vi "AI@Export2COCO__Parameter.vi"(1 "ParamterIn":string) -> (0 "ParamterOut":string)   [LabVIEW 2020]
uses:
  MainFrame/Global.vi
  <vilib>/vision/NI_Vision_Development_Module.lvlib
panel:
  out "start":i32
  out "f":i32
  in  "CoCoFile":string(combo)
  out "Image":T1(plugin-control)
  in  "Preview":bool
  in  "SubDir":string(combo)
  in  "Capture":string(combo)
  in  "Confirm":bool
  # "AI@Export2COCO $Capture(\\$Directory),$CoCo.json"
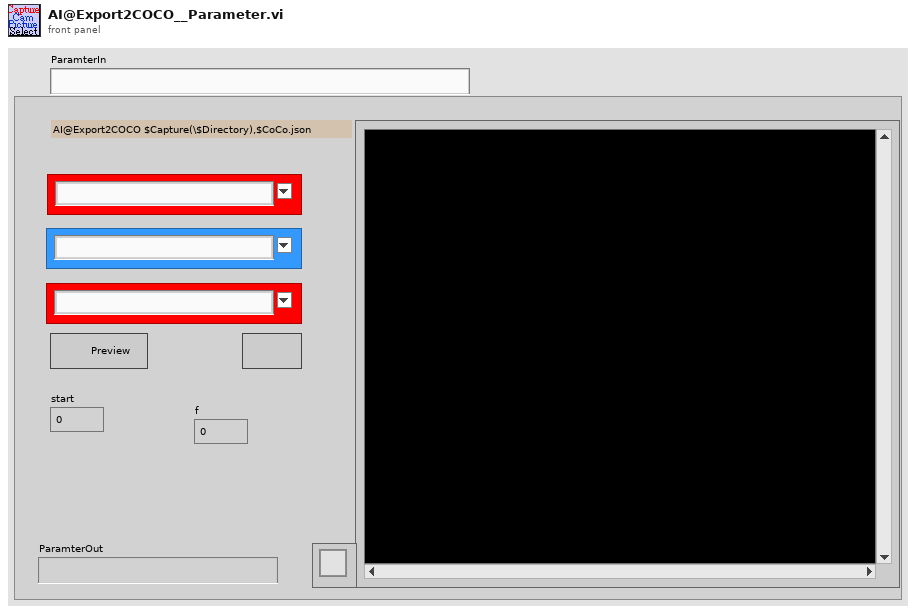
[diagram p1: front panel]
types:
  T1 = typedef "IMAQ Image.ctl" = refnum<image>
  T2 = cluster{"Browser Size":cluster{"X":i32, "Y":i32}, "Images per Line":i32, "Background Color":u32, "Frame Size":i32, "Frame Style":u16}
  T3 = typedef "Image Type" = u32
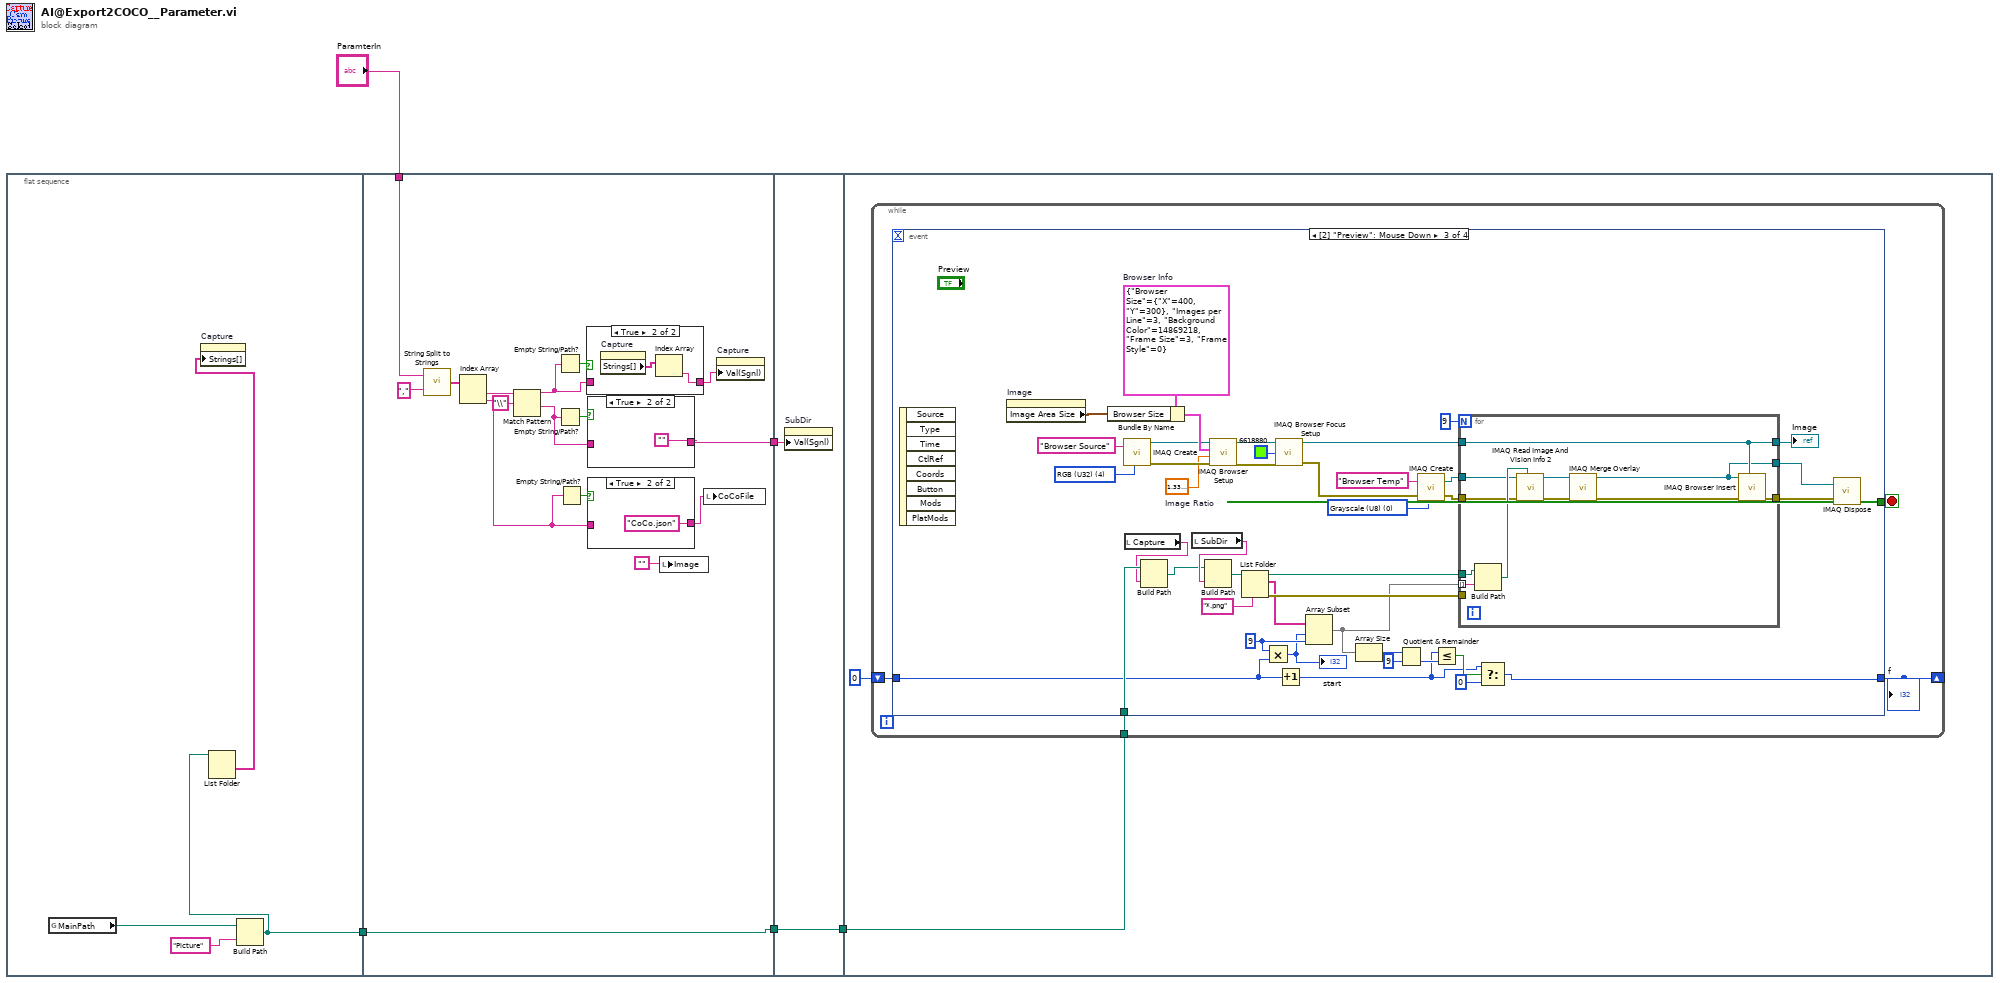
[diagram p0: block diagram]
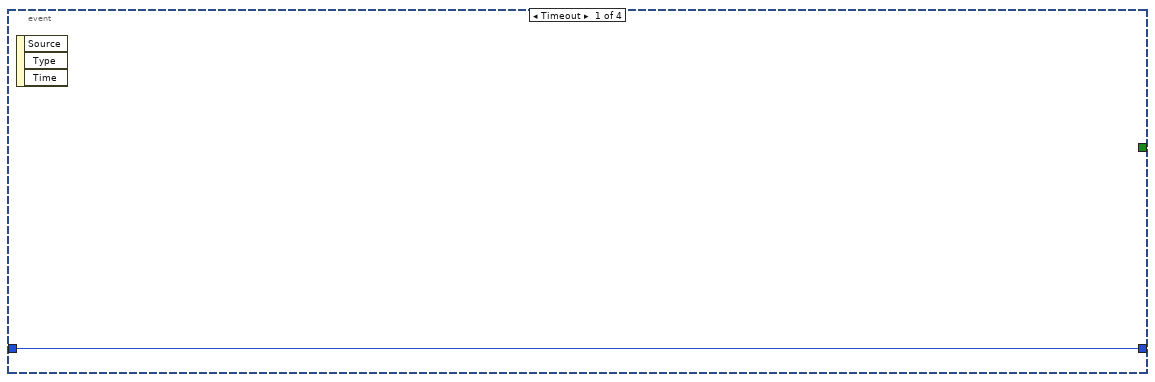
[diagram p5: hidden frame]
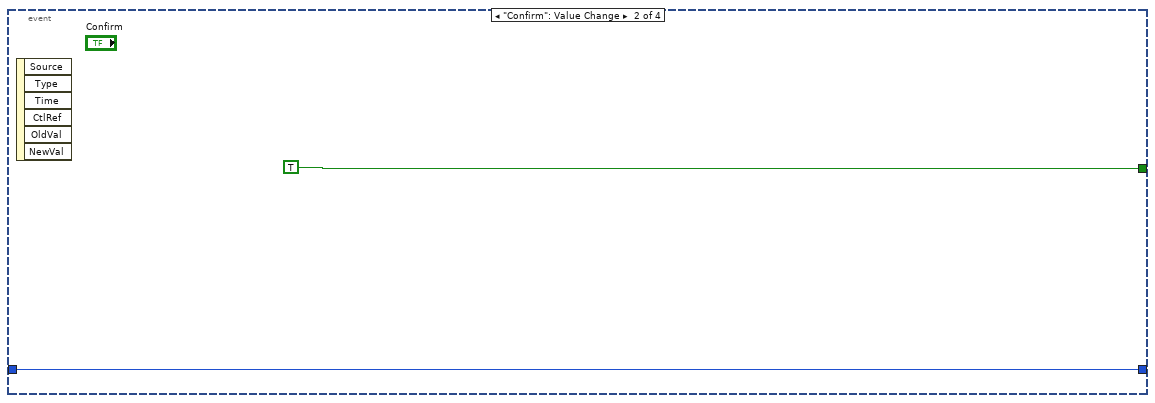
[diagram p6: hidden frame]
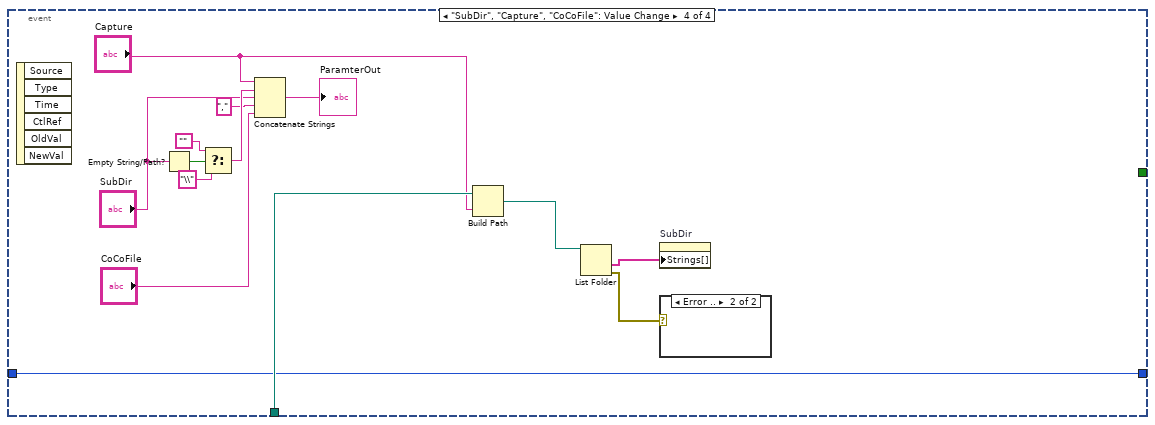
[diagram p7: hidden frame]
diagram:
  n1 = flat-sequence {
    tunnel: [w7] -> w2
    tunnel: "ParamterIn" -> [w23]
    tunnel: [w21] -> w3
    tunnel: w2 -> [w21]
    tunnel: [w20] -> w1
    tunnel: [w34] -> w4
    tunnel: w3 -> [w34]
    tunnel: w1 -> [w33]
    tunnel: w4 -> [w36]
    frame #0 {
      n2 = global read "Global.vi" "MainPath"() -> (w8:path)
      n3 = Build Path(base path=w8, name or relative path="Picture") -> (appended path=w7:path)
      n4 = List Folder(path=w7) -> (folder names=w6:string[])  [unwired: 3 in, 3 out]
      n5 = property on="Capture" class="CmbBox"("Strings[]"=w6) -> ()  [unwired: 2 in, 2 out]
    }
    frame #1 {
      n6 = call "String Split to Strings.vi"("search string/char (-)"=",", "String"=w23) -> ("Array"=w25:string[])
      n7 = Index Array(array=w25) -> (element #1=w17:string, element #2=w10:string)  [unwired: 2 in]
      n8 = Match Pattern(string=w17, regular expression="\\") -> (before substring=w15:string, after substring=w14:string)  [unwired: 1 in, 2 out]
      n9 = Empty String/Path?(string/path=w15) -> (empty?=w22:bool)
      n10 = Empty String/Path?(string/path=w14) -> (empty?=w18:bool)
      n11 = Empty String/Path?(string/path=w10) -> (empty?=w11:bool)
      n12 = case shown="True" w22 {
        tunnel: w15 -> [w30 _]
        tunnel: [w30 w31] -> w19
        frame False {
        }
        frame True {
          n13 = property on="Capture" class="CmbBox"() -> ("Strings[]"=w32:string[])  [unwired: 2 in, 2 out]
          n14 = Index Array(array=w32) -> (element=w31:string)  [unwired: 1 in]
        }
      }
      n15 = case shown="True" w18 {
        tunnel: [w28 ""] -> w20
        tunnel: w14 -> [w28 _]
        frame False {
        }
        frame True {
        }
      }
      n16 = case shown="True" w11 {
        tunnel: [w26 "CoCo.json"] -> w12
        tunnel: w10 -> [w26 _]
        frame False {
        }
        frame True {
        }
      }
      n17 = local write "Image"("") -> ()
      n18 = local write "CoCoFile"(w12) -> ()
      n19 = property on="Capture" class="CmbBox"("Val(Sgnl)"=w19) -> ()  [unwired: 2 in, 2 out]
    }
    frame #2 {
      n20 = property on="SubDir" class="CmbBox"("Val(Sgnl)"=w33) -> ()  [unwired: 2 in, 2 out]
    }
    frame #3 {
      n21 = while {
        tunnel: w36 -> [w39]
        shift-right: [w37] -> _
        shift-left: 0 -> [w38]
        stop <- w40 stop-if-true
        n22 = event shown="[2] \"Preview\": Mouse Down" {
          selector: _ -> [_ _ _ _]
          dyn-events: _ -> [_ _ _ _]
          timeout: _ -> [_ _ _ _]
          tunnel: [_ TRUE _ _] -> w40
          tunnel: w39 -> [_ _ w59 w107]
          tunnel: w38 -> [w41 w42 w53 w96]
          tunnel: [w41 w42 w45 w96] -> w37
          event Timeout {
            n23 = event-data() -> ()  [unwired: 1 in, 3 out]
          }
          event "Confirm": Value Change {
            n24 = event-data() -> ()  [unwired: 1 in, 6 out]
          }
          event "Preview": Mouse Down {
            w55 = 9 ("length")
            w63 = sgl 1.33  # Image Ratio
            w80 = T2 {"Browser Size"={"X"=400, "Y"=300}, "Images per Line"=3, "Background Color"=14869218, "Frame Size"=3, "Frame Style"=0}  # Browser Info
            w71 = T3 0 items=["Grayscale (U8)", "Grayscale (I16)", "Grayscale (SGL)", "Complex (CSG)", "RGB (U32)", "HSL (U32)", "RGB (U64)", "Grayscale (U16)"] ("Image Type")
            w69 = T3 4 items=["Grayscale (U8)", "Grayscale (I16)", "Grayscale (SGL)", "Complex (CSG)", "RGB (U32)", "HSL (U32)", "RGB (U64)", "Grayscale (U16)"] ("Image Type")
            n25 = event-data() -> ()  [unwired: 1 in, 8 out]
            n26 = property on="Image" class="ImageControl"() -> ("Image Area Size"=w81:cluster{"Width":u32, "Height":u32})  [unwired: 2 in, 2 out]
            n27 = Bundle By Name(cluster=w80, "Browser Size"=w81) -> (w82:T2)
            n28 = call "IMAQ Create"("Image Name"="Browser Source", "Image Type"=w69) -> ("New Image"=w67:T1, "error out"=w68:errorcluster)  [unwired: 3 in]
            n29 = local read "Capture"() -> (w58:string)
            n30 = Build Path(base path=w59, name or relative path=w58) -> (appended path=w57:path)
            n31 = local read "SubDir"() -> (w62:string)
            n32 = Build Path(base path=w57, name or relative path=w62) -> (appended path=w61:path)
            n33 = call "IMAQ Browser Setup"("error in (no error)"=w68, "Image Ratio"=w63, "Browser Info"=w82, "Image In"=w67) -> ("error out"=w76:errorcluster, "Image Browser Out"=w75:T1)  [unwired: 2 out]
            n34 = List Folder(path=w61, pattern="*.png") -> (path out=w66:path, filenames=w44:string[], error out=w83:errorcluster)  [unwired: 2 in, 1 out]
            n35 = Multiply(x=w55, y=w53) -> (x*y=w54:i32)
            "start" <- w54
            n36 = call "IMAQ Browser Focus Setup"("error in (no error)"=w76, "Focus Color"=u32 6618880, "Image Browser In"=w75) -> ("error out"=w78:errorcluster, "Image Browser Out"=w77:T1)  [unwired: 1 in]
            n37 = Increment(x=w53) -> (x+1=w47:i32)
            n38 = Array Subset(array=w44, index=w54, length=w55) -> (w52:string[])
            n39 = Array Size(array=w52) -> (size(s)=w51:i32)
            n40 = Quotient & Remainder(x=w51, y=9) -> (floor(x/y)=w49:i32)  [unwired: 1 out]
            n41 = call "IMAQ Create"("Image Name"="Browser Temp", "Image Type"=w71, "error in (no error)"=w78) -> ("New Image"=w73:T1, "error out"=w64:errorcluster)  [unwired: 2 in]
            n42 = Less Or Equal?(x=w47, y=w49) -> (x <= y?=w48:bool)
            n43 = for {
              N: 9 -> [_]
              tunnel: w77 -> [w90]
              tunnel: w66 -> [w95]
              tunnel: w64 -> [w93]
              tunnel: [w92] -> w65
              tunnel: [w90] -> w84
              tunnel: w73 -> [w91]
              tunnel: [w87] -> w74
              tunnel: w83 -> [_]
              tunnel: w52 -> [w85] mode=indexing
              n44 = Build Path(base path=w95, name or relative path=w85) -> (appended path=w94:path)
              n45 = call "IMAQ Read Image And Vision Info 2"("File Path"=w94, "error in (no error)"=w93, "Image"=w91) -> ("error out"=w89:errorcluster, "Image Out"=w88:T1)  [unwired: 6 in, 1 out]
              n46 = call "IMAQ Merge Overlay"("error in (no error)"=w89, "Image Src"=w88) -> ("error out"=w86:errorcluster, "Image Dst Out"=w87:T1)  [unwired: 8 in]
              n47 = call "IMAQ Browser Insert"("Image Browser In"=w90, "error in (no error)"=w86, "Image to Add"=w87) -> ("error out"=w92:errorcluster)  [unwired: 4 in, 4 out]
            }
            "Image" <- w84
            n48 = Select(t=w47, s=w48, f=0) -> (s? t:f=w45:i32)
            n49 = call "IMAQ Dispose"("Image"=w74, "error in (no error)"=w65) -> ()  [unwired: 4 in, 1 out]
          }
          event "SubDir", "Capture", "CoCoFile": Value Change {
            n50 = event-data() -> ()  [unwired: 1 in, 6 out]
            n51 = Empty String/Path?(string/path="SubDir") -> (empty?=w103:bool)
            n52 = Select(t="", s=w103, f="\\" ("string")) -> (s? t:f=w100:string)
            n53 = Concatenate Strings("Capture", w100, "SubDir", "," ("string"), "CoCoFile") -> (→"ParamterOut":string)
            n54 = Build Path(base path=w107, name or relative path="Capture") -> (appended path=w106:path)
            n55 = List Folder(path=w106) -> (folder names=w105:string[], error out=w108:errorcluster)  [unwired: 3 in, 2 out]
            n56 = property on="SubDir" class="CmbBox"("Strings[]"=w105) -> ()  [unwired: 2 in, 2 out]
            n57 = case shown="Error .." w108 {
              frame No Error {
              }
              frame Error {
              }
            }
          }
        }
        "f" <- w37
      }
    }
  }
